vi "Joystick to Swerve New.vi"(1 "Joystick R":dbl, 2 "Joystick X":dbl, 3 "Joystick Y":dbl) -> (0 "Swerve Data":T1)   [LabVIEW 2018]
uses:
  <vilib>/Rock Robotics/Network Tables/NT Write Boolean.vi
panel:
  out "D":dbl
  out "C":dbl
  out "B":dbl
  out "A":dbl
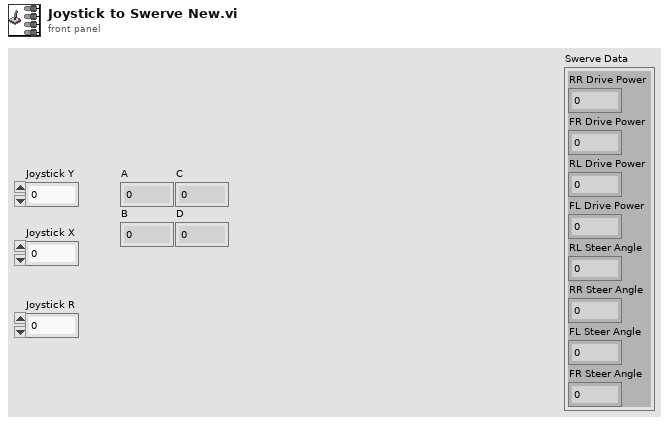
[diagram p1: front panel]
types:
  T1 = cluster{"RR Drive Power":dbl, "FR Drive Power":dbl, "RL Drive Power":dbl, "FL Drive Power":dbl, "RL Steer Angle":dbl, "RR Steer Angle":dbl, "FL Steer Angle":dbl, "FR Steer Angle":dbl}
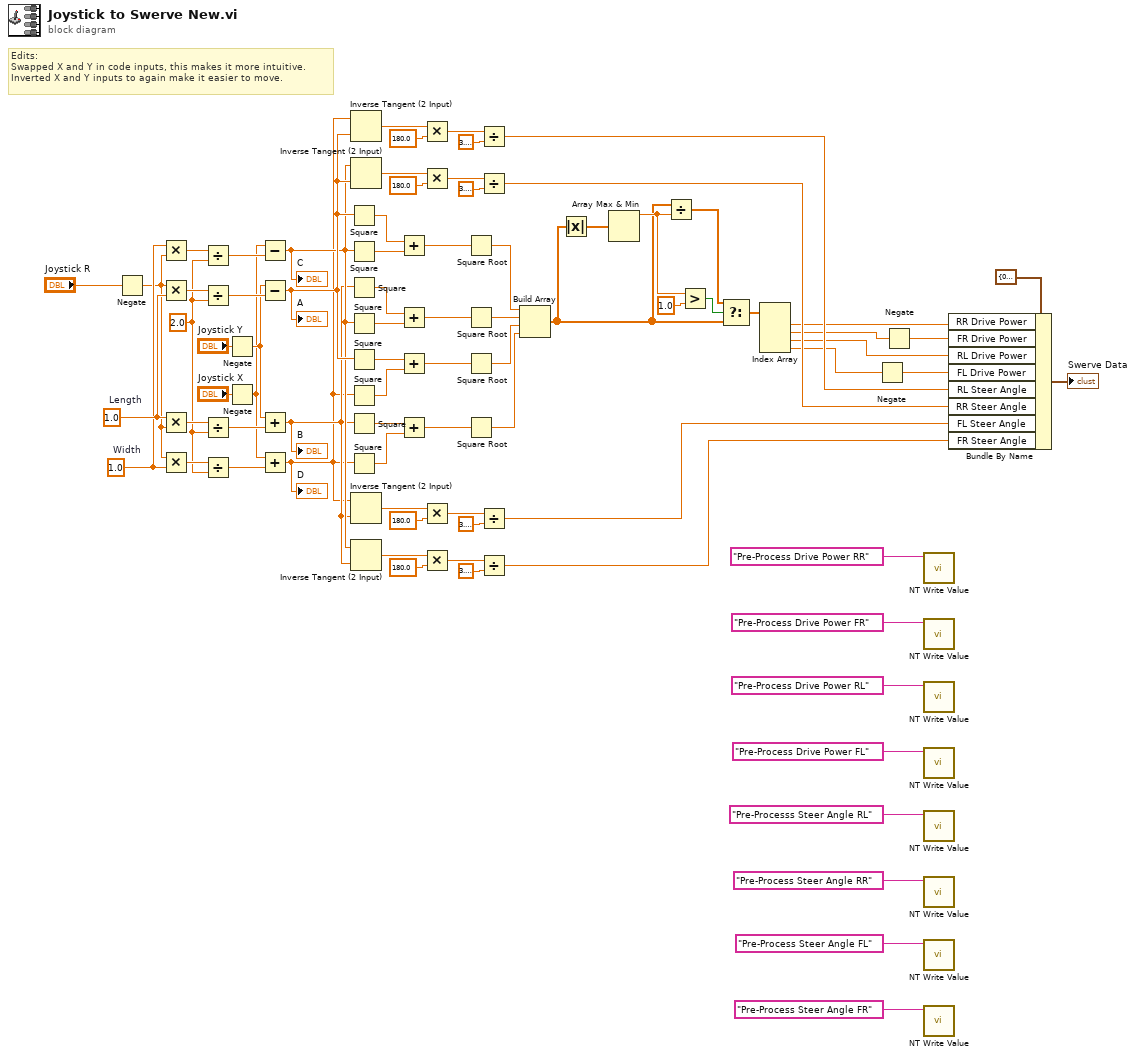
[diagram p0: block diagram]
diagram:
  w39 = 2.0
  w40 = 1.0  # Width
  w77 = 1.0  # Length
  # "Edits:\nSwapped X and Y in code inputs, this makes it more intuitive.\nInverted X and Y inputs to again make it easier to move."
  n1 = Negate(x="Joystick R") -> (-x=w34:dbl)
  n2 = Multiply(x=w40, y=w34) -> (x*y=w74:dbl)
  n3 = Multiply(x=w34, y=w77) -> (x*y=w80:dbl)
  n4 = Multiply(x=w77, y=w34) -> (x*y=w76:dbl)
  n5 = Multiply(x=w34, y=w40) -> (x*y=w71:dbl)
  n6 = Divide(x=w74, y=w39) -> (x/y=w73:dbl)
  n7 = Divide(x=w80, y=w39) -> (x/y=w79:dbl)
  n8 = Divide(x=w76, y=w39) -> (x/y=w75:dbl)
  n9 = Divide(x=w71, y=w39) -> (x/y=w70:dbl)
  n10 = Negate(x="Joystick Y") -> (-x=w14:dbl)
  n11 = Negate(x="Joystick X") -> (-x=w13:dbl)
  n12 = Subtract(x=w13, y=w73) -> (x-y=w37:dbl)
  "C" <- w37
  n13 = Subtract(x=w14, y=w79) -> (x-y=w38:dbl)
  "A" <- w38
  n14 = Add(x=w14, y=w75) -> (x+y=w36:dbl)
  "B" <- w36
  n15 = Add(x=w13, y=w70) -> (x+y=w35:dbl)
  "D" <- w35
  n16 = Square(x=w38) -> (x^2=w44:dbl)
  n17 = Square(x=w37) -> (x^2=w43:dbl)
  n18 = Square(x=w36) -> (x^2=w65:dbl)
  n19 = Square(x=w37) -> (x^2=w64:dbl)
  n20 = Square(x=w38) -> (x^2=w51:dbl)
  n21 = Square(x=w35) -> (x^2=w50:dbl)
  n22 = Square(x=w36) -> (x^2=w58:dbl)
  n23 = Square(x=w35) -> (x^2=w57:dbl)
  n24 = Inverse Tangent (2 Input)(1:w38, 2:w35) -> (0:w55:dbl)
  n25 = Inverse Tangent (2 Input)(1:w38, 2:w37) -> (0:w48:dbl)
  n26 = Inverse Tangent (2 Input)(1:w36, 2:w35) -> (0:w62:dbl)
  n27 = Inverse Tangent (2 Input)(1:w36, 2:w37) -> (0:w69:dbl)
  n28 = Add(x=w44, y=w43) -> (x+y=w42:dbl)
  n29 = Add(x=w65, y=w64) -> (x+y=w63:dbl)
  n30 = Add(x=w51, y=w50) -> (x+y=w49:dbl)
  n31 = Add(x=w58, y=w57) -> (x+y=w56:dbl)
  n32 = Multiply(x=w55, y=180.0) -> (x*y=w52:dbl)
  n33 = Multiply(x=w48, y=180.0) -> (x*y=w46:dbl)
  n34 = Multiply(x=w62, y=180.0) -> (x*y=w59:dbl)
  n35 = Multiply(x=w69, y=180.0) -> (x*y=w66:dbl)
  n36 = Square Root(x=w42) -> (sqrt(x)=w33:dbl)
  n37 = Square Root(x=w63) -> (sqrt(x)=w32:dbl)
  n38 = Square Root(x=w49) -> (sqrt(x)=w31:dbl)
  n39 = Square Root(x=w56) -> (sqrt(x)=w30:dbl)
  n40 = Divide(x=w52, y=3.141592653589793) -> (x/y=w22:dbl)
  n41 = Divide(x=w46, y=3.141592653589793) -> (x/y=w21:dbl)
  n42 = Divide(x=w59, y=3.141592653589793) -> (x/y=w20:dbl)
  n43 = Divide(x=w66, y=3.141592653589793) -> (x/y=w17:dbl)
  n44 = Build Array(w33, w32, w31, w30) -> (w24:dbl[])
  n45 = Absolute Value(x=w24) -> (abs(x)=w29:dbl[])
  n46 = Array Max & Min(array=w29) -> (max value=w26:dbl)  [unwired: 3 out]
  n47 = Divide(x=w24, y=w26) -> (x/y=w25:dbl[])
  n48 = Greater?(x=w26, y=1.0) -> (0:w27:bool)
  n49 = Select(t=w25, s=w27, f=w24) -> (s? t:f=w23:dbl[])
  n50 = Index Array(array=w23) -> (element #1=w12:dbl, element #2=w11:dbl, element #3=w10:dbl, element #4=w9:dbl)  [unwired: 4 in]
  n51 = Negate(x=w9) -> (-x=w15:dbl)
  n52 = Negate(x=w11) -> (-x=w16:dbl)
  n53 = call-poly <vilib>:"NT Write Value.vi"("Name"="Pre-Process Drive Power RR") -> ()  [unwired: 10 in, 1 out]
  n54 = call-poly <vilib>:"NT Write Value.vi"("Name"="Pre-Process Drive Power FR") -> ()  [unwired: 10 in, 1 out]
  n55 = call-poly <vilib>:"NT Write Value.vi"("Name"="Pre-Process Drive Power RL") -> ()  [unwired: 10 in, 1 out]
  n56 = call-poly <vilib>:"NT Write Value.vi"("Name"="Pre-Process Drive Power FL") -> ()  [unwired: 10 in, 1 out]
  n57 = call-poly <vilib>:"NT Write Value.vi"("Name"="Pre-Processs Steer Angle RL") -> ()  [unwired: 10 in, 1 out]
  n58 = call-poly <vilib>:"NT Write Value.vi"("Name"="Pre-Process Steer Angle RR") -> ()  [unwired: 10 in, 1 out]
  n59 = call-poly <vilib>:"NT Write Value.vi"("Name"="Pre-Process Steer Angle FL") -> ()  [unwired: 10 in, 1 out]
  n60 = call-poly <vilib>:"NT Write Value.vi"("Name"="Pre-Process Steer Angle FR") -> ()  [unwired: 10 in, 1 out]
  n61 = Bundle By Name(cluster=T1 {"RR Drive Power"=0.0, "FR Drive Power"=0.0, "RL Drive Power"=0.0, "FL Drive Power"=0.0, "RL Steer Angle"=0.0, "RR Steer Angle"=0.0, "FL Steer Angle"=0.0, "FR Steer Angle"=0.0}, "RR Drive Power"=w12, "FR Drive Power"=w16, "RL Drive Power"=w10, "FL Drive Power"=w15, "RL Steer Angle"=w22, "RR Steer Angle"=w21, "FL Steer Angle"=w20, "FR Steer Angle"=w17) -> (→"Swerve Data":T1)
